vi "5.PID-Host GUI DataLog.vi"() -> ()   [LabVIEW 2014]
doc: "This example demonstrates how to implement a STM client which receives messages from the server.\n\nThe server needs to be started before the client."
uses:
  vi.lib/Q-WaveSystems/QwaveSys Raspberry Pi for LabVIEW Home-Education/STM/TCP/STM Read Meta Data (TCP Ref).vi
  <vilib>/Utility/file.llb/Write To Spreadsheet File (DBL).vi
  vi.lib/Q-WaveSystems/QwaveSys Raspberry Pi for LabVIEW Home-Education/STM/TCP/STM Read Message (TCP).vi
  vi.lib/Q-WaveSystems/QwaveSys Raspberry Pi for LabVIEW Home-Education/STM/TCP/STM Get Connection Reference (TCP).vi
  vi.lib/Q-WaveSystems/QwaveSys Raspberry Pi for LabVIEW Home-Education/QwaveSys Raspberry Pi Library.lvlib
panel:
  out "Output (MV)":dbl(graph)
  out "Alarm Higher Limit":bool
  out "Alarm Lower Limit":bool
  out "Max":dbl
  out "Min":dbl
  out "SP":dbl
  out "PV":dbl
  out "Monitor Chart":cluster{"initial PV":dbl, "SP:":dbl, dbl, dbl}(graph)
  out "error  out":errorcluster
  in  "Target IP Address":string="192.168.5.1"
  in  "stop":bool
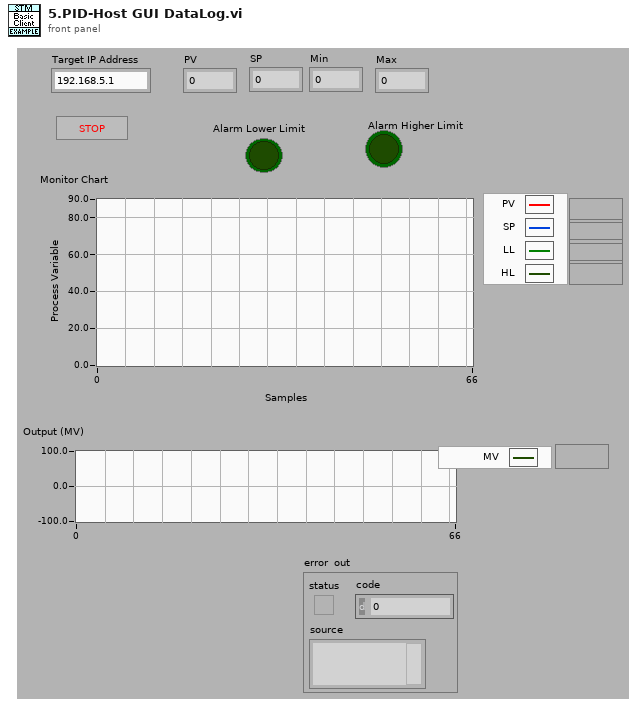
[diagram p1: front panel]
types:
  T1 = typedef "QwaveSys Raspberry Pi Library.lvlib/stm_TCP Connection Info.ctl" = cluster{"connection ID":refnum<k5>, "Meta data":T2[]}
  T2 = typedef "QwaveSys Raspberry Pi Library.lvlib/stm_MetaDataElement.ctl" = string
  T3 = cluster{"PV":dbl, "SP":dbl, "Min":dbl, "Max":dbl}
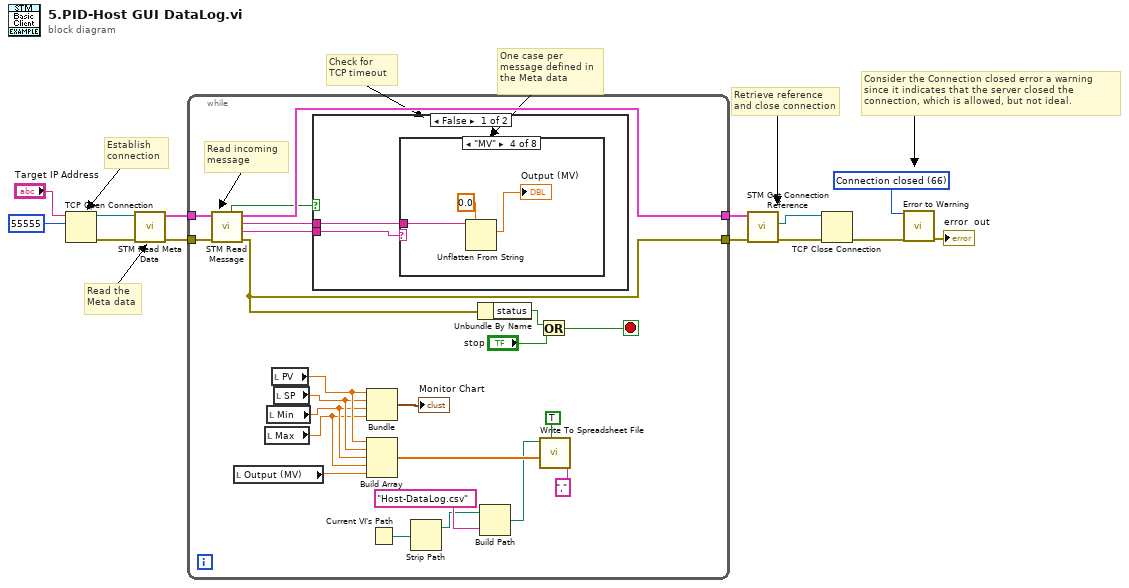
[diagram p0: block diagram]
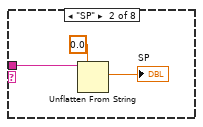
[diagram p3: hidden frame]
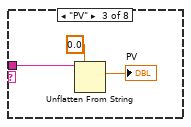
[diagram p4: hidden frame]
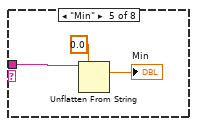
[diagram p5: hidden frame]
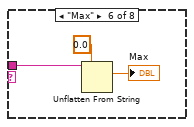
[diagram p6: hidden frame]
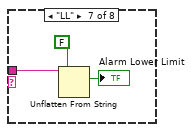
[diagram p7: hidden frame]
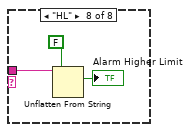
[diagram p8: hidden frame]
diagram:
  w7 = 66 items=["No Error", "Argument Error", "Memory Full", "Out of Zone", "End of File", "File Already Open", "Generic File IO Error", "File Not Found", "File Permission Error", "Disk Full", "Duplicate Path", "Too Many Files Open", "Not Enabled", "Resource File Not Found", "Cannot Add Resource", "Resource Not Found", "Image Not Found", "Image Memory Error", "Pen Does Not Exist", "Config Bad Type", "Config Token Not Found", "Config Parse Error", "Config Memory Error", "Bad External Code Format", "Bad External Code Offset", "External Code Not Present", "Null Window", "Destroy Window Mixup", "Null Menu", "Print Aborted", "Bad Print Record", "Print Driver Error", "Windows Error During Print", "Memory Error During Print", "Print Dialog Error", "Generic Print Error", "Invalid Device Refnum", "Device Not Found", "Device Parameter Error", "Device Unit Error", "Can't Open Device", "Device Call Aborted", "Generic Error", "Cancelled By User", "Object ID Too Low", "Object ID Too High", "Object Not In Heap", "Unknown Heap", "Bad DefProc ID", "DefProc Not In Table", "Message Out Of Range", "Null Method", "Unknown Message", "Manager Call Not Supported", "Bad address", "Connection In progress", "Connection timed out", "Connection is already in progress", "Network attribute not supported", "Network error", "Address in use", "System out of memory", "Connection aborted", "Connection refused", "Connection is not connected", "Connection is already connected", "Connection closed", "Initialize error (interapplication manager)", "Bad occurrence", "Wait on unbound occurrence handler", "Occurrence queue overflow", "Bad path", "Semaphore not signaled", "Unrecognized type (interapplication manager)"] ("1st Error to Convert")
  # "Consider the Connection closed error a warning since it indicates that the server closed the connection, which is allowed, but not ideal."
  # "Retrieve reference and close connection"
  # "Check for\nTCP timeout"
  # "One case per\nmessage defined in\nthe Meta data"
  # "Read the \nMeta data"
  # "Establish\nconnection"
  n1 = TCP Open Connection(address="Target IP Address", remote port or service name=u16 55555 ("remote port")) -> (connection ID=w13:refnum<k5>, error out=w11:errorcluster)  [unwired: 1 in, 2 out]
  n2 = call-poly "STM Read Meta Data.vi"("error in"=w11, "connection ID"=w13) -> ("error out"=w10:errorcluster, "Connection Info Out"=w12:T1)  [unwired: 1 in, 7 out]
  n3 = while {
    tunnel: w12 -> [w36]
    tunnel: w10 -> [w35]
    tunnel: [w34] -> w4
    tunnel: [w31] -> w3
    stop <- w28 stop-if-true
    # "Read incoming\nmessage"
    n4 = call-poly "STM Read Message.vi"("error in"=w35, "Connection Info"=w36) -> ("error out"=w31:errorcluster, "Name"=w33:T2, "data string"=w32:string, "Connection Info Out"=w34:T1, "Timed Out?"=w27:bool)  [unwired: 1 in, 4 out]
    n5 = local read "Output (MV)"() -> (w16:dbl)
    n6 = local read "Max"() -> (w17:dbl)
    n7 = local read "Min"() -> (w18:dbl)
    n8 = local read "PV"() -> (w20:dbl)
    n9 = local read "SP"() -> (w19:dbl)
    n10 = case shown="False" w27 {
      tunnel: w33 -> [w37 _]
      tunnel: w32 -> [w38 _]
      frame False {
        n11 = case shown="\"MV\"" w37 {
          tunnel: w38 -> [_ w39 w42 w46 w48 w51 w56 w59]
          frame Default {
          }
          frame "SP" {
            n12 = Unflatten From String(type=0.0, binary string=w39) -> (value=→"SP":dbl)  [unwired: 1 in, 4 out]
          }
          frame "PV" {
            n13 = Unflatten From String(type=0.0, binary string=w42) -> (value=→"PV":dbl)  [unwired: 1 in, 4 out]
          }
          frame "MV" {
            n14 = Unflatten From String(type=0.0, binary string=w46) -> (value=→"Output (MV)":dbl)  [unwired: 1 in, 4 out]
          }
          frame "Min" {
            n15 = Unflatten From String(type=0.0, binary string=w48) -> (value=→"Min":dbl)  [unwired: 1 in, 4 out]
          }
          frame "Max" {
            n16 = Unflatten From String(type=0.0, binary string=w51) -> (value=→"Max":dbl)  [unwired: 1 in, 4 out]
          }
          frame "LL" {
            n17 = Unflatten From String(type=FALSE, binary string=w56) -> (value=→"Alarm Lower Limit":bool)  [unwired: 1 in, 4 out]
          }
          frame "HL" {
            n18 = Unflatten From String(type=FALSE, binary string=w59) -> (value=→"Alarm Higher Limit":bool)  [unwired: 1 in, 4 out]
          }
        }
      }
      frame True {
      }
    }
    n19 = Bundle("PV"=w20, "SP"=w19, "Min"=w18, "Max"=w17) -> (→"Monitor Chart":T3)  [unwired: 1 in]
    n20 = Build Array(w20, w19, w18, w17, w16) -> (w15:dbl[])
    n21 = Current VI's Path() -> (path=w25:path)
    n22 = Strip Path(path=w25) -> (stripped path=w23:path)  [unwired: 1 out]
    n23 = Unbundle By Name(w31) -> ("status"=w30:bool)
    n24 = Build Path(base path=w23, name or relative path="Host-DataLog.csv") -> (appended path=w14:path)
    n25 = Or(x=w30, y="stop") -> (x .or. y?=w28:bool)
    n26 = call-poly <vilib>:"Write To Spreadsheet File.vi"("delimiter (\\t)"="," ("delimiter (\\t)"), "append to file? (new file:F)"=TRUE, "1D data"=w15, "file path (dialog if empty)"=w14) -> ()  [unwired: 4 in, 1 out]
  }
  n27 = call-poly "STM Get Connection Reference.vi"("error in"=w3, "Connection Info"=w4) -> ("error out"=w1:errorcluster, "connection ID out"=w2:refnum<k5>)  [unwired: 8 out]
  n28 = TCP Close Connection(connection ID=w2, error in (no error)=w1) -> (error out=w6:errorcluster)  [unwired: 2 out]
  n29 = call <vilib>:"Error to Warning.vi"("1st Error to Convert"=w7, "error in"=w6) -> ("warning out"=→"error  out":errorcluster)  [unwired: 3 in, 10 out]
